vi "LeerArchivoConfiguracion.vi"(8 "error in":errorcluster, 11 "Prueba31 in":refnum<class "Prueba03.lvclass">) -> (0 "error out":errorcluster, 3 "Prueba31 out":refnum<class "Prueba03.lvclass">)   [LabVIEW 2019, in "Prueba03.lvclass"]
uses:
  Prueba03.lvclass
  Prueba03.lvclass/Prueba03.ctl
  <vilib>/Utility/config.llb/Read Key (Boolean).vi
  <vilib>/Utility/config.llb/Read Key (String).vi
  <vilib>/Utility/config.llb/NI_LVConfig.lvlib
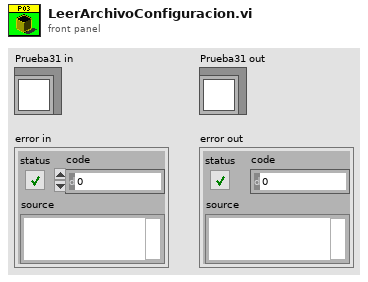
[diagram p1: front panel]
types:
  T1 = typedef "NI_LVConfig.lvlib/Config Data RefNum.ctl" = refnum<k1>
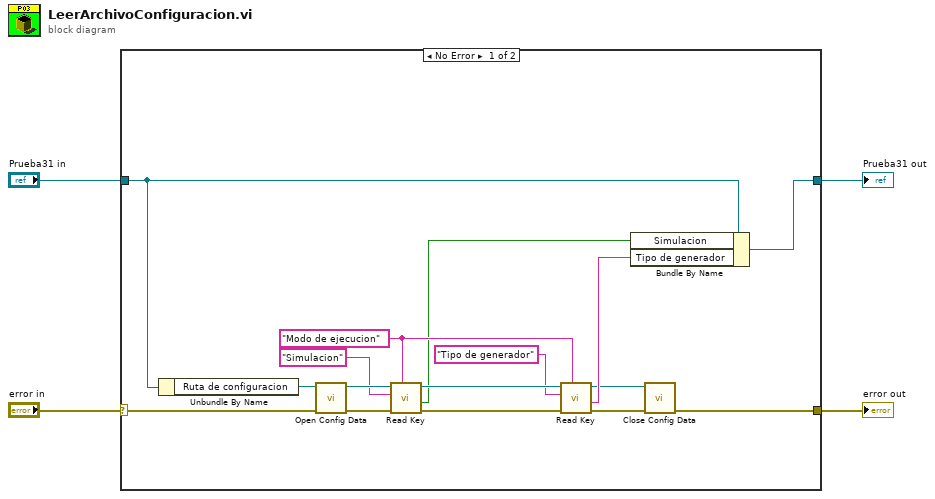
[diagram p0: block diagram]
diagram:
  n1 = case shown="No Error" "error in" {
    selector: "error in" -> [w20 w21]
    tunnel: [w8 w21] -> w2
    tunnel: [w6 w22] -> w4
    tunnel: "Prueba31 in" -> [w5 w22]
    frame No Error {
      w14 = "Modo de ejecucion" ("section")
      n2 = Unbundle By Name(w5) -> ("Ruta de configuracion"=w19:path)
      n3 = call <vilib>:"Open Config Data.vi"("error in (no error)"=w20, "configuration file path"=w19) -> ("error out"=w18:errorcluster, "refnum"=w17:T1)  [unwired: 7 in, 1 out]
      n4 = call-poly <vilib>:"Read Key.vi"("section"=w14, "error in (no error)"=w18, "key"="Simulacion", "refnum"=w17) -> ("error out"=w13:errorcluster, "value"=w12:bool, "refnum out"=w15:T1)  [unwired: 4 in, 1 out]
      n5 = call-poly <vilib>:"Read Key.vi"("section"=w14, "error in (no error)"=w13, "key"="Tipo de generador", "refnum"=w15) -> ("error out"=w9:errorcluster, "value"=w10:string, "refnum out"=w7:T1)  [unwired: 4 in, 1 out]
      n6 = Bundle By Name(cluster=w5, "Simulacion"=w12, "Tipo de generador"=w10) -> (w6:refnum<class "Prueba03.lvclass">)
      n7 = call <vilib>:"Close Config Data.vi"("error in (no error)"=w9, "refnum"=w7) -> ("error out"=w8:errorcluster)  [unwired: 8 in, 1 out]
    }
    frame Error {
    }
  }
  "Prueba31 out" <- w4
  "error out" <- w2
